vi "setAddress.vi"(8 "error in (no error)":errorcluster, 10 "Address":u8, 11 "FrameBuilder in":refnum<class "DynamicFrameBuilder.lvclass">) -> (0 "error out":errorcluster, 3 "FrameBuilder out":refnum<class "DynamicFrameBuilder.lvclass">)   [LabVIEW 2015, in "RTModbus.lvlib" / "DynamicFrameBuilder.lvclass"]
uses:
  DynamicFrameBuilder.lvclass
  DynamicFrameBuilder.lvclass/DynamicFrameBuilder.ctl
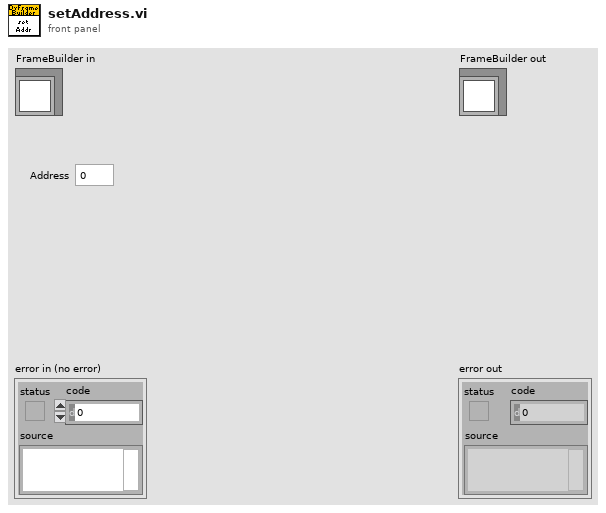
[diagram p1: front panel]
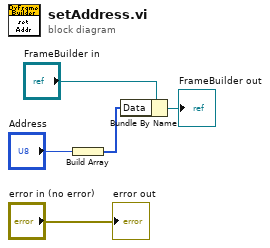
[diagram p0: block diagram]
diagram:
  n1 = Build Array("Address") -> (w3:u8[])
  n2 = Bundle By Name(cluster="FrameBuilder in", "Data"=w3) -> (→"FrameBuilder out":refnum<class "DynamicFrameBuilder.lvclass">)
  "error out" <- "error in (no error)"
